vi "getLocalQueueType.vi"() -> (3 "Queue Type":refnum<queue>)   [LabVIEW 2013, in "MQTT_Queue.lvlib" / "LocalQueueConnection.lvclass"]
uses:
  LocalQueueConnection.lvclass
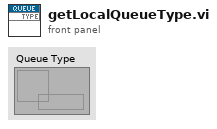
[diagram p1: front panel]
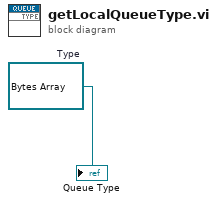
[diagram p0: block diagram]
diagram:
  w1 = refnum<queue> refnum  # Type
  "Queue Type" <- w1
